vi "Pump read and get mode.vi"(0 "VISA resource name":refnum<visa-resource-name>="COM1", 5 "Address (00)":i32 format="%02.0f", 11 "error in (no error)":errorcluster) -> (4 "VISA resource name out":refnum<visa-resource-name>, 8 "Output String":string, 10 "Pump status":T1 items=["Error - Can't read status"=-1, "Stopped"=0, "Infusing"=1, "Withdrawing"=2, "Pump stalled"=3, "Stopped at infuse limit"=4, "Stopped at withdraw limit"=5, "Emergency stop"=6, "Stopped at target volume"=7], 15 "error out":errorcluster)   [LabVIEW 2015]
doc: "Reads a response from the pump affter a command is sent\n\nModified from original which is Copyright 2005, National Instruments Corporation"
uses:
  Pump status.ctl
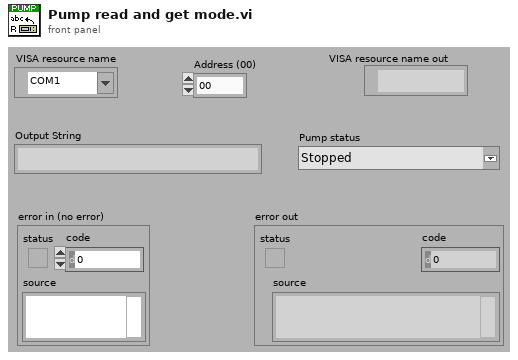
[diagram p1: front panel]
types:
  T1 = typedef "Pump status.ctl" = i8
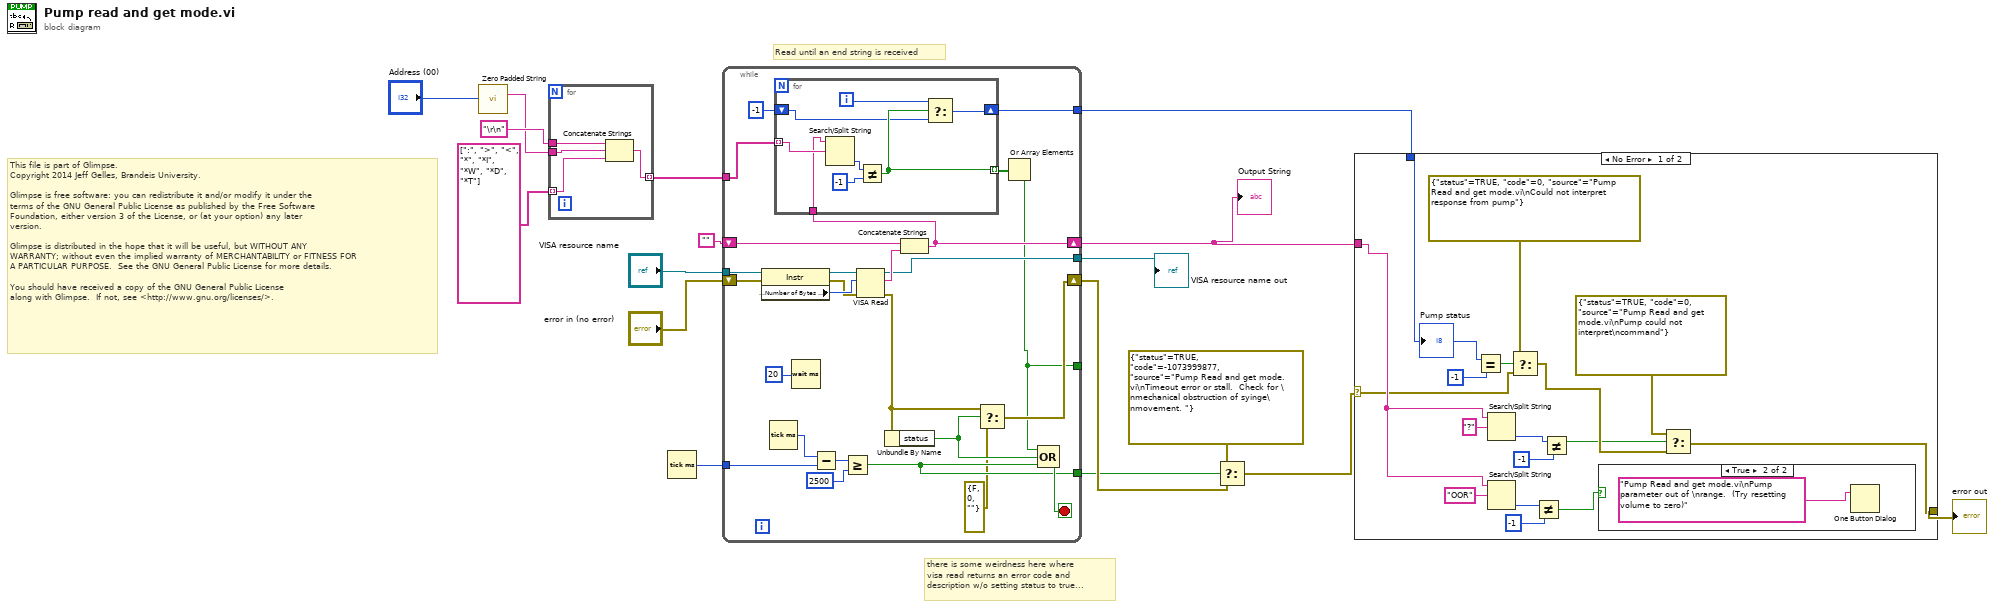
[diagram p0: block diagram]
diagram:
  # "This file is part of Glimpse. \nCopyright 2014 Jeff Gelles, Brandeis University.    \n\nGlimpse is free software: you can redistribute it and/or modify it under the \nterms of the GNU General Public License as published by the Free Software \nFoundation, either version 3 of the License, or (at your option) any later \nversion.\n\nGlimpse is distributed in the hope that it will be useful, but WITHOUT ANY \nWARRANTY; without even the implied warranty of MERCHANTABILITY or FITNESS FOR \nA PARTICULAR PURPOSE.  See the GNU General Public License for more details.\n\nYou should have received a copy of the GNU General Public License\nalong with Glimpse.  If not, see <http://www.gnu.org/licenses/>."
  # "there is some weirdness here where \nvisa read returns an error code and\ndescription w/o setting status to true..."
  # "Read until an end string is received"
  n1 = call "Zero Padded String.vi"("Address (00)"="Address (00)") -> ("Zero Padded Address String"=w3:string)  [unwired: 14 out]
  n2 = for {
    tunnel: string[] [":", ">", "<", "*", "*I", "*W", "*D", "*T"] ("string array") -> [w19] mode=indexing
    tunnel: "\r\n" -> [w21]
    tunnel: w3 -> [w20]
    tunnel: [w18] -> w6 mode=indexing
    n3 = Concatenate Strings(w21, w20, w19) -> (w18:string)
  }
  n4 = Tick Count (ms)() -> (millisecond timer value=w14:u32)
  n5 = while {
    tunnel: "VISA resource name" -> [w46]
    shift-right: [w27] -> w9
    shift-left: "" -> [w40]
    tunnel: [w39] -> w11
    tunnel: w14 -> [w36]
    tunnel: [w32] -> w2
    tunnel: [w24] -> _
    shift-right: [w28] -> w13
    shift-left: "error in (no error)" -> [w42]
    tunnel: w6 -> [w26]
    tunnel: [w22] -> w5
    stop <- w33 stop-if-true
    n6 = property class="Instr"(reference=w46, error in=w42) -> (reference out=w44:refnum<visa-resource-name>, error out=w43:errorcluster, "Serial Settings:Number of Bytes at Serial Port"=w45:u32)
    n7 = Tick Count (ms)() -> (millisecond timer value=w37:u32)
    n8 = Wait (ms)(milliseconds to wait=u32 20) -> ()  [unwired: 1 out]
    n9 = Subtract(x=w37, y=w36) -> (x-y=w35:u32)
    n10 = Greater Or Equal?(x=w35, y=u32 2500) -> (x >= y?=w32:bool)
    n11 = VISA Read(VISA resource name=w44, byte count=w45, error in (no error)=w43) -> (VISA resource name out=w39:refnum<visa-resource-name>, read buffer=w41:string, error out=w30:errorcluster)  [unwired: 1 out]
    n12 = Unbundle By Name(w30) -> ("status"=w31:bool)
    n13 = Concatenate Strings(w40, w41) -> (w27:string)
    n14 = for {
      tunnel: w27 -> [w47]
      tunnel: w26 -> [w48] mode=indexing
      tunnel: [w51] -> w25 mode=indexing
      shift-right: [w52] -> w22
      shift-left: -1 -> [w50]
      i -> [w49]
      n15 = Search/Split String(string=w47, search string/char (-)=w48) -> (offset of match=w53:i32)  [unwired: 3 out]
      n16 = Not Equal?(x=w53, y=-1) -> (x != y?=w51:bool)
      n17 = Select(t=w49, s=w51, f=w50) -> (s? t:f=w52:i32)
    }
    n18 = Select(t=w30, s=w31, f=errorcluster {"status"=FALSE, "code"=0, "source"=""}) -> (s? t:f=w28:errorcluster)
    n19 = Or Array Elements(Boolean array=w25) -> (logical OR=w24:bool)
    n20 = Compound Arithmetic op=OR(w24, w31, w32) -> (w33:bool)
  }
  "Output String" <- w9
  "VISA resource name out" <- w11
  n21 = Select(t=errorcluster {"status"=TRUE, "code"=-1073999877, "source"="Pump Read and get mode.vi\nTimeout error or stall.  Check for \nmechanical obstruction of syinge\nmovement. "}, s=w2, f=w13) -> (s? t:f=w10:errorcluster)
  n22 = case shown="No Error" w10 {
    selector: w10 -> [w59 w73]
    tunnel: w9 -> [w71 _]
    tunnel: [w56 w73] -> w1
    tunnel: w5 -> [w57 _]
    frame No Error {
      n23 = Equal?(x=w57, y=-1) -> (x = y?=w60:bool)
      n24 = Search/Split String(string=w71, search string/char (-)="?") -> (offset of match=w65:i32)  [unwired: 3 out]
      n25 = Search/Split String(string=w71, search string/char (-)="OOR") -> (offset of match=w66:i32)  [unwired: 3 out]
      n26 = Select(t=errorcluster {"status"=TRUE, "code"=0, "source"="Pump Read and get mode.vi\nCould not interpret response from pump"}, s=w60, f=w59) -> (s? t:f=w63:errorcluster)
      n27 = Not Equal?(x=w66, y=-1) -> (x != y?=w55:bool)
      n28 = Not Equal?(x=w65, y=-1) -> (x != y?=w58:bool)
      n29 = case shown="True" w55 {
        frame False {
        }
        frame True {
          n30 = One Button Dialog(message="Pump Read and get mode.vi\nPump parameter out of \nrange.  (Try resetting volume to zero)" ("source")) -> ()  [unwired: 2 out]
        }
      }
      n31 = Select(t=errorcluster {"status"=TRUE, "code"=0, "source"="Pump Read and get mode.vi\nPump could not interpret\ncommand"}, s=w58, f=w63) -> (s? t:f=w56:errorcluster)
      "Pump status" <- w57
    }
    frame Error {
    }
  }
  "error out" <- w1
